vi "Generate Signal Block.vi"(4 "amplitude":dbl=1.0, 5 "frequency":dbl=10.0, 6 "sample rate":dbl=1000.0, 7 "noise level":dbl, 8 "error in":errorcluster, 9 "signal type":enum32{"Sine", "Square", "Chirp"}(ring), 10 "start sample":dbl, 11 "samples":i32=100) -> (0 "error out":errorcluster, 1 "time":dbl[](array[numeric]), 2 "signal":dbl[](array[numeric]), 3 "next start sample":dbl)   [LabVIEW 2026, in "Signal Generator.lvlib"]
doc: "Signal generation engine. Computes one contiguous block of a synthetic waveform (sine, square or linear chirp) with additive uniform noise, starting at an absolute sample index so consecutive blocks join without a phase discontinuity. Amplitude is the peak value, frequency is in Hz, sample rate in S/s and noise level is the RMS noise amplitude. A chirp sweeps from frequency up to min(10 x frequency, 0.45 x sample rate) in one second and repeats."
uses:
  Signal Generator.lvlib
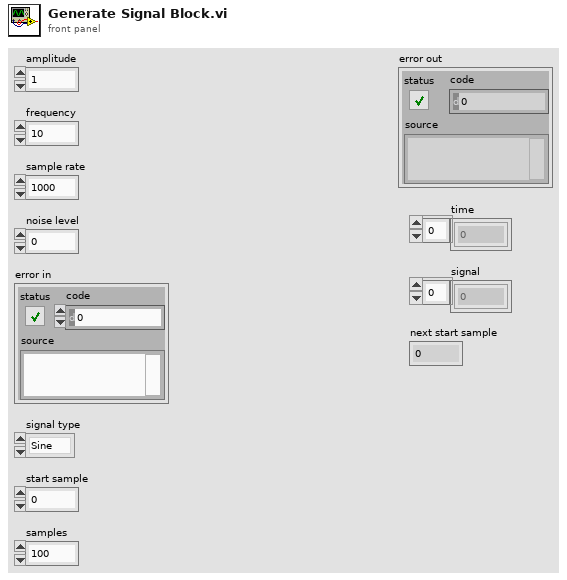
[diagram p1: front panel]
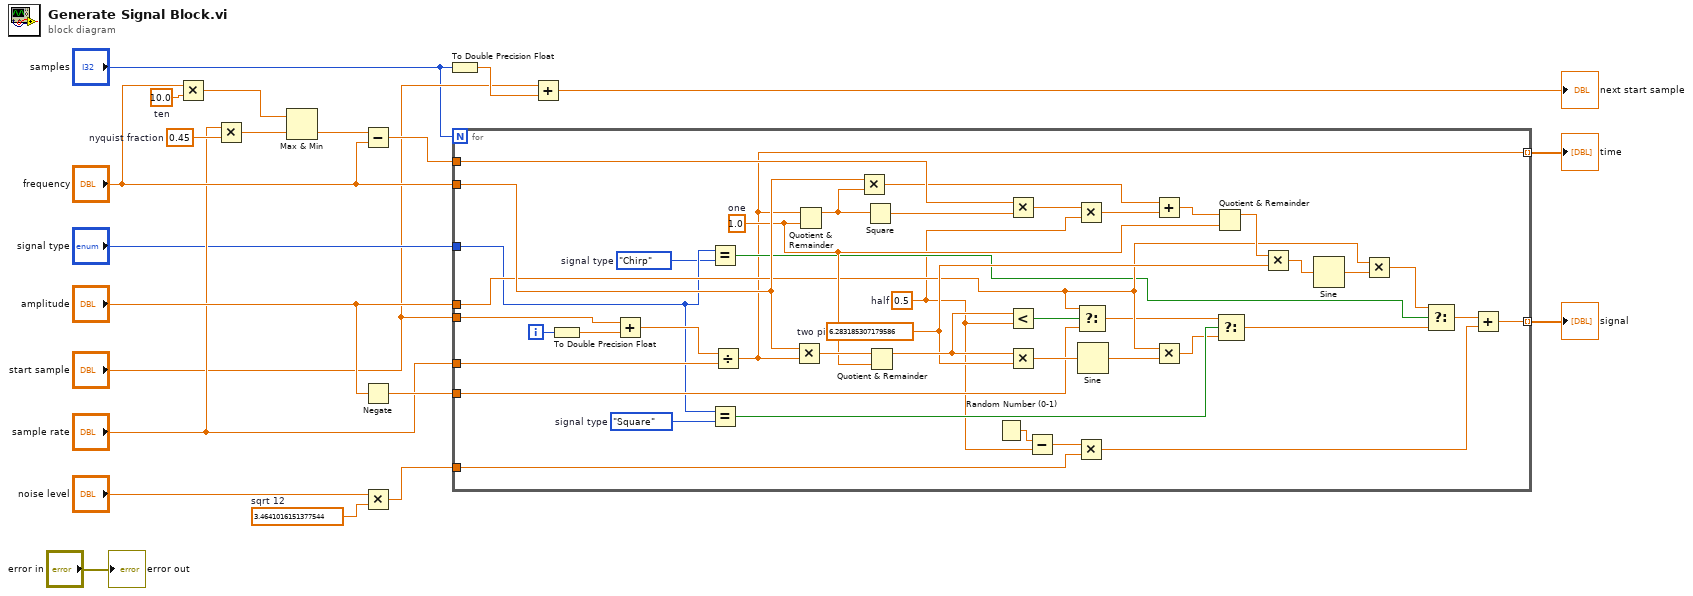
[diagram p0: block diagram]
diagram:
  w15 = 3.4641016151377544  # sqrt 12
  w20 = 0.45  # nyquist fraction
  w21 = 10.0  # ten
  n1 = Multiply(x="frequency", y=w21) -> (x*y=w19:dbl)
  n2 = Multiply(x="sample rate", y=w20) -> (x*y=w18:dbl)
  n3 = Max & Min(x=w19, y=w18) -> (min(x,y)=w17:dbl)  [unwired: 1 out]
  n4 = Subtract(x=w17, y="frequency") -> (x-y=w9:dbl)
  n5 = Negate(x="amplitude") -> (-x=w12:dbl)
  n6 = Multiply(x="noise level", y=w15) -> (x*y=w8:dbl)
  n7 = To Double Precision Float(number="samples") -> (double precision float=w14:dbl)
  n8 = for {
    N: "samples" -> [_]
    tunnel: "amplitude" -> [w41]
    tunnel: w12 -> [w54]
    tunnel: "frequency" -> [w53]
    tunnel: "sample rate" -> [w60]
    tunnel: w9 -> [w51]
    tunnel: w8 -> [w27]
    tunnel: "signal type" -> [w38]
    tunnel: "start sample" -> [w63]
    tunnel: [w24] -> w3 mode=indexing
    tunnel: [w23] -> w2 mode=indexing
    i -> [w22]
    w37 = enum32{"Sine", "Square", "Chirp"}."Chirp"  # signal type
    w39 = enum32{"Sine", "Square", "Chirp"}."Square"  # signal type
    w43 = 6.283185307179586  # two pi
    w29 = 0.5  # half
    w45 = 1.0  # one
    n9 = To Double Precision Float(number=w22) -> (double precision float=w62:dbl)
    n10 = Add(x=w63, y=w62) -> (x+y=w61:dbl)
    n11 = Equal?(x=w38, y=w37) -> (x = y?=w32:bool)
    n12 = Equal?(x=w38, y=w39) -> (x = y?=w35:bool)
    n13 = Divide(x=w61, y=w60) -> (x/y=w24:dbl)
    n14 = Multiply(x=w53, y=w24) -> (x*y=w59:dbl)
    n15 = Quotient & Remainder(x=w24, y=w45) -> (x-y*floor(x/y)=w52:dbl)  [unwired: 1 out]
    n16 = Multiply(x=w53, y=w52) -> (x*y=w48:dbl)
    n17 = Square(x=w52) -> (x^2=w50:dbl)
    n18 = Quotient & Remainder(x=w59, y=w45) -> (x-y*floor(x/y)=w56:dbl)  [unwired: 1 out]
    n19 = Random Number (0-1)() -> (number: 0 to 1=w30:dbl)
    n20 = Multiply(x=w51, y=w50) -> (x*y=w49:dbl)
    n21 = Less?(x=w56, y=w29) -> (x < y?=w55:bool)
    n22 = Multiply(x=w56, y=w43) -> (x*y=w58:dbl)
    n23 = Subtract(x=w30, y=w29) -> (x-y=w28:dbl)
    n24 = Multiply(x=w49, y=w29) -> (x*y=w47:dbl)
    n25 = Multiply(x=w28, y=w27) -> (x*y=w25:dbl)
    n26 = Select(t=w41, s=w55, f=w54) -> (s? t:f=w36:dbl)
    n27 = Sine(x=w58) -> (sin(x)=w57:dbl)
    n28 = Add(x=w48, y=w47) -> (x+y=w46:dbl)
    n29 = Multiply(x=w41, y=w57) -> (x*y=w34:dbl)
    n30 = Quotient & Remainder(x=w46, y=w45) -> (x-y*floor(x/y)=w44:dbl)  [unwired: 1 out]
    n31 = Select(t=w36, s=w35, f=w34) -> (s? t:f=w31:dbl)
    n32 = Multiply(x=w44, y=w43) -> (x*y=w42:dbl)
    n33 = Sine(x=w42) -> (sin(x)=w40:dbl)
    n34 = Multiply(x=w41, y=w40) -> (x*y=w33:dbl)
    n35 = Select(t=w33, s=w32, f=w31) -> (s? t:f=w26:dbl)
    n36 = Add(x=w26, y=w25) -> (x+y=w23:dbl)
  }
  "time" <- w3
  "signal" <- w2
  n37 = Add(x="start sample", y=w14) -> (x+y=→"next start sample":dbl)
  "error out" <- "error in"
